vi "Invert Current Keithley 220.vi"(2 "Point #":i32, 5 "Instrument Address":refnum<visa-resource-name>) -> (0 "Stop":bool, 1 "Keithley 220 Current":dbl[](array[numeric]) format="%.2e")   [LabVIEW 2019]
doc: "VI to reverse the current for a Keithley 220 current source to be able to take a running average of voltages and remove any constant EMFs in the leads.\nScott Hannahs, NHMF, Jan 1995"
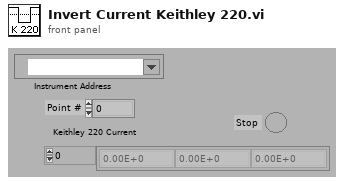
[diagram p1: front panel]
types:
  T1 = cluster{"Instrument":string, "ID Test String":string, "Terminator Character":string, u32, bool}
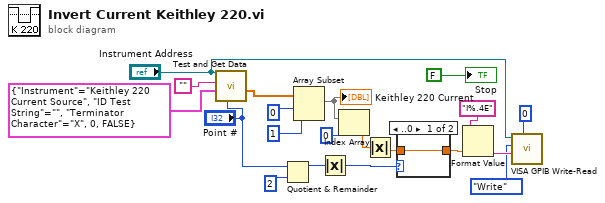
[diagram p0: block diagram]
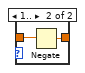
[diagram p2: hidden frame]
diagram:
  n1 = call "Test and Get Data.vi"("Point #"="Point #", "Instrument Info"=T1 {"Instrument"="Keithley 220 Current Source", "ID Test String"="", "Terminator Character"="X", 0, FALSE}, "Command String"="", "VISA Sesson"="Instrument Address") -> ("Measurement"=w5:dbl[])  [unwired: 2 in, 4 out]
  n2 = Quotient & Remainder(x="Point #", y=2) -> (x-y*floor(x/y)=w17:i32)  [unwired: 1 out]
  n3 = Array Subset(array=w5, index=0, length=1) -> (w8:dbl[])
  "Keithley 220 Current" <- w8
  n4 = Absolute Value(x=w17) -> (abs(x)=w9:i32)
  n5 = Index Array(array=w8, index=0) -> (element=w12:dbl)
  n6 = Absolute Value(x=w12) -> (abs(x)=w11:dbl)
  n7 = case shown="..0" w9 {
    tunnel: [w21 w23] -> w18
    tunnel: w11 -> [w21 w22]
    frame ..0 {
    }
    frame 1.. {
      n8 = Negate(x=w22) -> (-x=w23:dbl)
    }
  }
  n9 = Format Value(format string="I%.4E", value (0)=w18) -> (output string=w7:string)  [unwired: 1 in]
  n10 = call "VISA GPIB Write-Read.vi"("Wait (ms)"=u32 0, "Command"=w7, "Action"=enum16{"Write", "Read", "Write & Read"}."Write", "VISA resource name"="Instrument Address") -> ()  [unwired: 4 in, 4 out]
  "Stop" <- FALSE
